vi "Replace Array Elements [DBL].vi"(9 "Array of Replacement Pairs":cluster{"Original":dbl, "New":dbl}[](array[cluster]), 11 "Array":dbl[](array[numeric])) -> (3 "Array with Replacements":dbl[](array[numeric]))   [LabVIEW 2019]
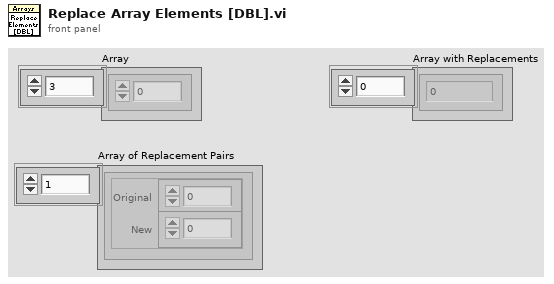
[diagram p1: front panel]
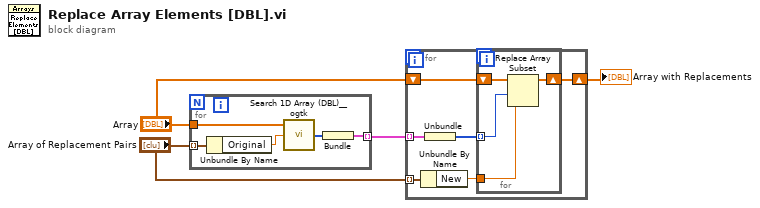
[diagram p0: block diagram]
diagram:
  n1 = for {
    tunnel: "Array of Replacement Pairs" -> [w8] mode=indexing
    tunnel: "Array" -> [w9]
    tunnel: [w5] -> w3 mode=indexing
    n2 = Unbundle By Name(w8) -> ("Original"=w7:dbl)
    n3 = call <userlib>:"Search 1D Array (DBL)__ogtk.vi"("Array"=w9, "Element Data"=w7) -> ("Indices of Elements"=w6:i32[])  [unwired: 7 in]
    n4 = Bundle("Indices of Elements"=w6) -> (w5:cluster{"Indices of Elements":i32[]})  [unwired: 1 in]
  }
  n5 = for {
    tunnel: "Array of Replacement Pairs" -> [w15] mode=indexing
    tunnel: w3 -> [w14] mode=indexing
    shift-right: [w12] -> w1
    shift-left: "Array" -> [w13]
    n6 = Unbundle By Name(w15) -> ("New"=w10:dbl)
    n7 = Unbundle(w14) -> ("Indices of Elements"=w11:i32[])
    n8 = for {
      shift-right: [w16] -> w12
      shift-left: w13 -> [w19]
      tunnel: w11 -> [w18] mode=indexing
      tunnel: w10 -> [w17]
      n9 = Replace Array Subset(array=w19, new element=w17, index=w18) -> (w16:dbl[])
    }
  }
  "Array with Replacements" <- w1
